vi "读地址转报文.vi"(10 "读取触点类型":string, 11 "读取起始地址":string) -> (3 "连接的字符串":string)   [LabVIEW 2018]
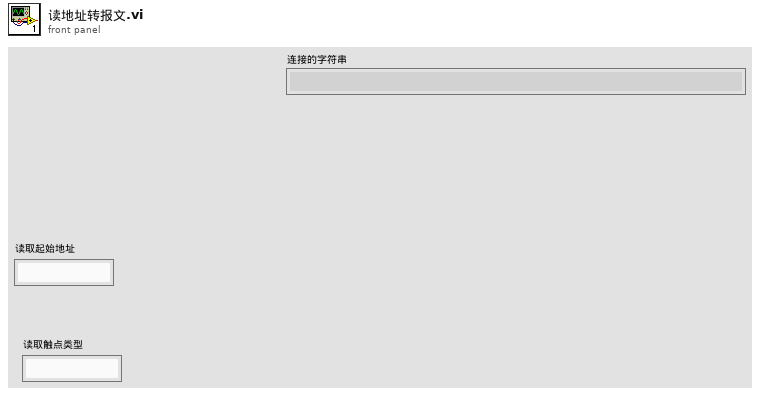
[diagram p1: front panel]
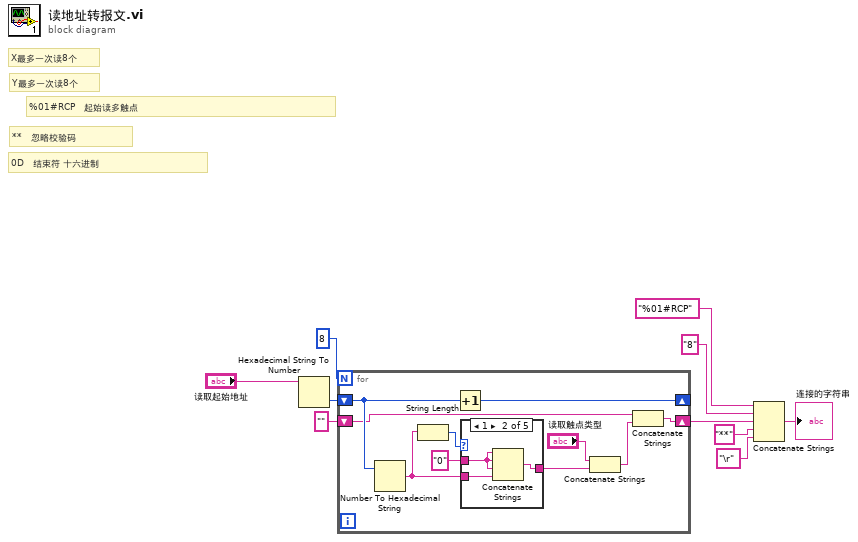
[diagram p0: block diagram]
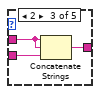
[diagram p3: hidden frame]
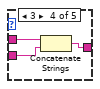
[diagram p4: hidden frame]
diagram:
  # "Y最多一次读8个"
  # "X最多一次读8个"
  # "0D   结束符 十六进制"
  # "**   忽略校验码"
  # "%01#RCP   起始读多触点"
  n1 = Hexadecimal String To Number(string="读取起始地址") -> (number=w1:u32)  [unwired: 2 in, 1 out]
  n2 = for {
    N: 8 -> [_]
    shift-right: [w20] -> _
    shift-left: w1 -> [w19]
    shift-right: [w12] -> w4
    shift-left: "" -> [w14]
    n3 = Number To Hexadecimal String(2:w19) -> (0:w17:string)  [unwired: 1 in]
    n4 = String Length(string=w17) -> (length=w18:i32)
    n5 = Increment(x=w19) -> (x+1=w20:u32)
    n6 = case shown="1" w18 {
      tunnel: w17 -> [w21 w23 w26 w29 w31]
      tunnel: "0" -> [_ w24 w27 w30 _]
      tunnel: [w21 w22 w25 w28 w31] -> w15
      frame 0, Default {
      }
      frame 1 {
        n7 = Concatenate Strings(w24, w24, w24, w23) -> (w22:string)
      }
      frame 2 {
        n8 = Concatenate Strings(w27, w27, w26) -> (w25:string)
      }
      frame 3 {
        n9 = Concatenate Strings(w30, w29) -> (w28:string)
      }
      frame 4 {
      }
    }
    n10 = Concatenate Strings("读取触点类型", w15) -> (w13:string)
    n11 = Concatenate Strings(w14, w13) -> (w12:string)
  }
  n12 = Concatenate Strings("%01#RCP" ("字符串"), "8" ("字符串"), w4, "**" ("字符串"), "\r" ("字符串")) -> (→"连接的字符串":string)
